vi "Puff_using_Arduino.vi"() -> (5 "Plug in titles":string[](array[string]), 7 "Plug in values":string[](array[string]))   [LabVIEW 2013]
uses:
  Controls/Post_Process.ctl
  Controls/Setup.ctl
  Globals/Meas_global.vi
panel:
  out "Puff Time used":dbl=1.0 format="%.2g"
  out "EnFlo_Tunnel Metadata:Puff_duration:Sec":dbl=1.0 format="%.2g"
  out "Case Currently On":string="Loop"
  # "Change this value via the ADAM Scan Table"
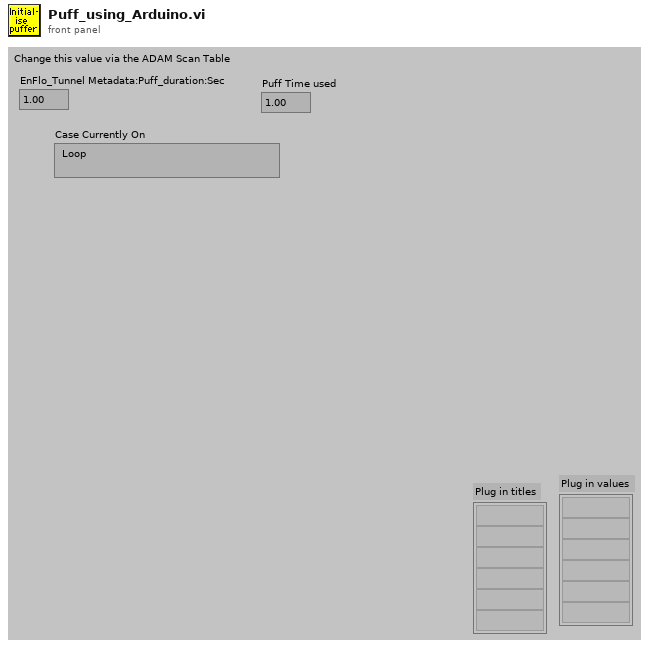
[diagram p1: front panel]
types:
  T1 = typedef "Setup.ctl" = enum16{"Run Program", "Show Setup", "Save Current Setup", "Setup Front Panel"}
  T2 = typedef "Post_Process.ctl" = enum16{"Take New Data", "Post Process Raw Data File"}
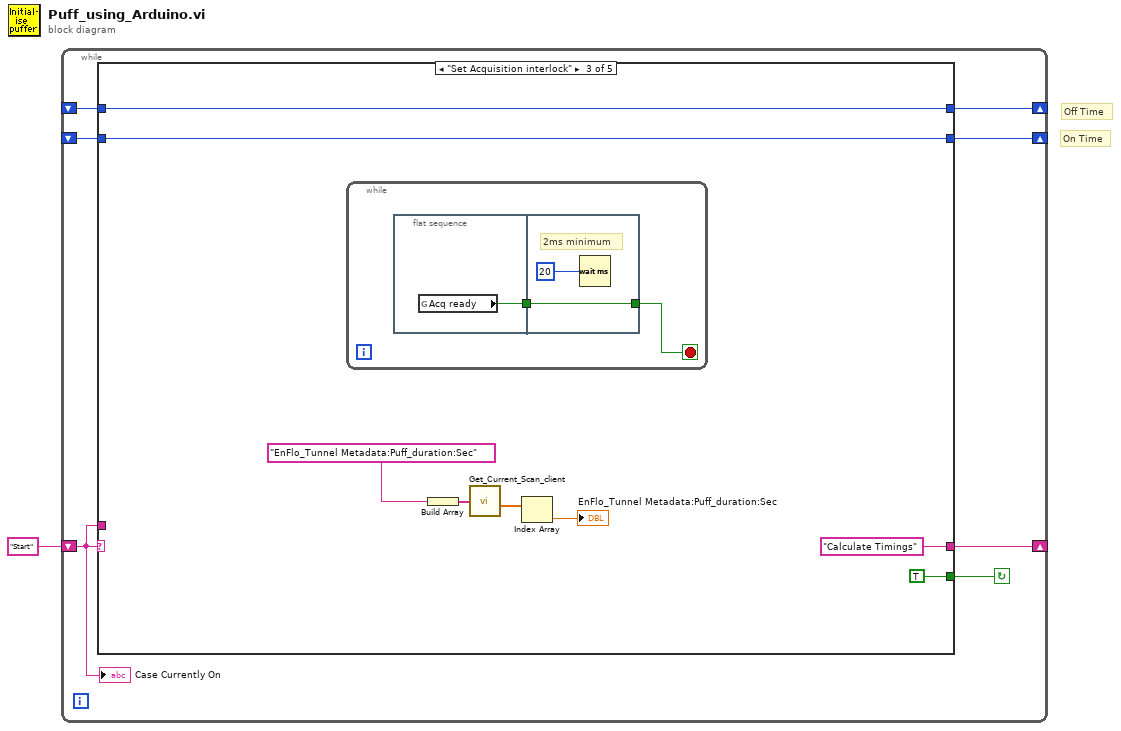
[diagram p0: block diagram]
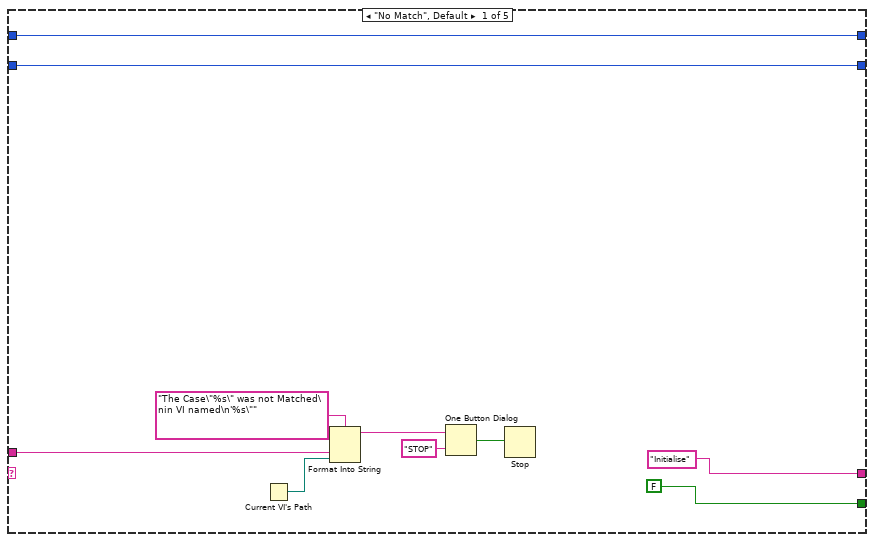
[diagram p2: hidden frame]
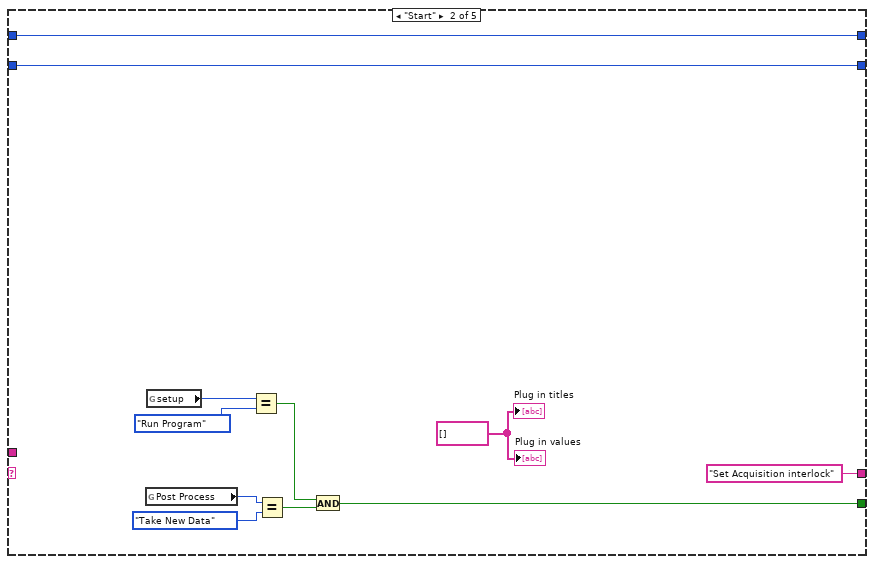
[diagram p3: hidden frame]
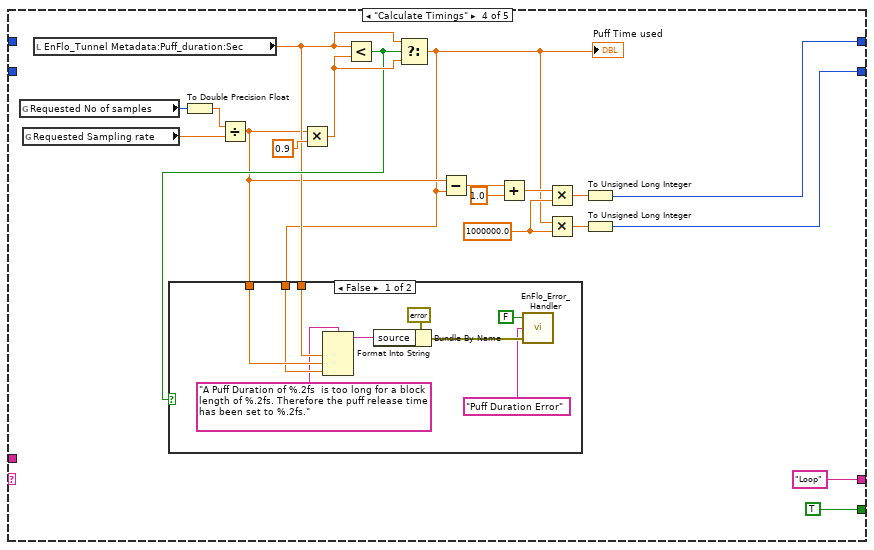
[diagram p4: hidden frame]
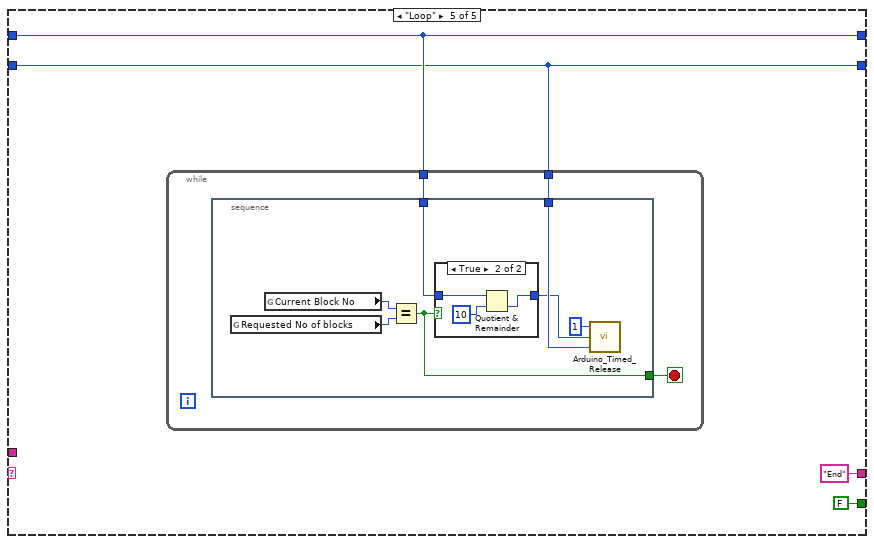
[diagram p6: hidden frame]
diagram:
  # "On Time"
  # "Off Time"
  n1 = while {
    shift-left: "Start" -> [w6]
    shift-right: [w7] -> _
    shift-right: [w5] -> _
    shift-left: _ -> [w4]
    shift-right: [w3] -> _
    shift-left: _ -> [w2]
    stop <- w8 continue-if-true
    n2 = case shown="\"Set Acquisition interlock\"" w6 {
      tunnel: [FALSE w21 TRUE ("Command Found") TRUE ("Command Found") FALSE ("Command Found")] -> w8
      tunnel: ["Initialise" "Set Acquisition interlock" "Calculate Timings" "Loop" "End"] -> w7
      tunnel: w6 -> [w13 _ _ _ _]
      tunnel: [w10 w20 w31 w45 w74] -> w5
      tunnel: w4 -> [w10 w20 w31 _ w74]
      tunnel: [w9 w19 w30 w44 w73] -> w3
      tunnel: w2 -> [w9 w19 w30 _ w73]
      frame "No Match", Default {
        n3 = Current VI's Path() -> (path=w12:path)
        n4 = Format Into String(format string="The Case\"%s\" was not Matched\nin VI named\n'%s\"" ("Format String"), w13, w12) -> (resulting string=w16:string)  [unwired: 2 in, 1 out]
        n5 = One Button Dialog(message=w16, button name ("OK")="STOP") -> (true=w14:bool)
        n6 = Stop(stop? (T)=w14) -> ()
      }
      frame "Start" {
        w28 = string[] [] ("Plug in titles")
        n7 = global read "Meas_global.vi" "Post Process"() -> (w23:T2)
        n8 = global read "Meas_global.vi" "setup"() -> (w22:T1)
        n9 = Equal?(x=w22, y=Setup."Run Program") -> (x = y?=w27:bool)
        n10 = Equal?(x=w23, y=Post_Process."Take New Data" ("Post Process")) -> (x = y?=w26:bool)
        n11 = And(x=w27, y=w26) -> (x .and. y?=w21:bool)
        "Plug in values" <- w28
        "Plug in titles" <- w28
      }
      frame "Set Acquisition interlock" {
        n12 = while {
          stop <- w39 stop-if-true
          n13 = flat-sequence {
            tunnel: [w40] -> w38
            tunnel: [w42] -> w39
            tunnel: w38 -> [w42]
            frame #0 {
              n14 = global read "Meas_global.vi" "Acq ready"() -> (w40:bool)
            }
            frame #1 {
              # "2ms minimum"
              n15 = Wait (ms)(milliseconds to wait=u32 20) -> ()  [unwired: 1 out]
            }
          }
        }
        n16 = Build Array("EnFlo_Tunnel Metadata:Puff_duration:Sec") -> (w34:string[])
        n17 = call "Get_Current_Scan_client.vi"("ADAM Ch Names"=w34) -> ("Numerical Values"=w33:dbl[])  [unwired: 1 in, 2 out]
        n18 = Index Array(array=w33) -> (element=→"EnFlo_Tunnel Metadata:Puff_duration:Sec":dbl)  [unwired: 1 in]
      }
      frame "Calculate Timings" {
        w54 = 1000000.0 ("y")
        n19 = global read "Meas_global.vi" "Requested No of samples"() -> (w59:i32)
        n20 = global read "Meas_global.vi" "Requested Sampling rate"() -> (w48:dbl)
        n21 = local read "EnFlo_Tunnel Metadata:Puff_duration:Sec"() -> (w49:dbl)
        n22 = To Double Precision Float(number=w59) -> (double precision float=w43:dbl)
        n23 = Divide(x=w43, y=w48) -> (x/y=w47:dbl)
        n24 = Multiply(x=w47, y=0.9) -> (x*y=w57:dbl)
        n25 = Less?(x=w49, y=w57) -> (x < y?=w50:bool)
        n26 = Select(t=w49, s=w50, f=w57) -> (s? t:f=w46:dbl)
        "Puff Time used" <- w46
        n27 = case shown="False" w50 {
          tunnel: w49 -> [w68 _]
          tunnel: w47 -> [w67 _]
          tunnel: w46 -> [w66 _]
          frame False {
            n28 = Format Into String(format string="A Puff Duration of %.2fs  is too long for a block length of %.2fs. Therefore the puff release time has been set to %.2fs.", w68, w67, w66) -> (resulting string=w64:string)  [unwired: 2 in, 1 out]
            n29 = Bundle By Name(cluster=errorcluster {"status"=TRUE, "code"=0, "source"=""} ("error in (no error)"), "source"=w64) -> (w69:errorcluster)
            n30 = call "EnFlo_Error_Handler.vi"("error in (no error)"=w69, "Error Type"="Puff Duration Error", "Dialog Box (T)"=FALSE) -> ()  [unwired: 3 out]
          }
          frame True {
          }
        }
        n31 = Subtract(x=w47, y=w46) -> (x-y=w53:dbl)
        n32 = Add(x=w53, y=1.0) -> (x+y=w51:dbl)
        n33 = Multiply(x=w51, y=w54) -> (x*y=w55:dbl)
        n34 = Multiply(x=w46, y=w54) -> (x*y=w56:dbl)
        n35 = To Unsigned Long Integer(number=w55) -> (unsigned 32bit integer=w45:u32)
        n36 = To Unsigned Long Integer(number=w56) -> (unsigned 32bit integer=w44:u32)
      }
      frame "Loop" {
        n37 = while {
          tunnel: w74 -> [w75]
          tunnel: w73 -> [w77]
          stop <- w76 stop-if-true
          n38 = stacked-sequence {
            tunnel: w77 -> [w83]
            tunnel: [w78] -> w76
            tunnel: w75 -> [w82]
            frame #0 {
              n39 = global read "Meas_global.vi" "Requested No of blocks"() -> (w80:i32)
              n40 = global read "Meas_global.vi" "Current Block No"() -> (w79:i32)
              n41 = Equal?(x=w79, y=w80) -> (x = y?=w78:bool)
              n42 = case shown="True" w78 {
                tunnel: w82 -> [w85 w88]
                tunnel: [w85 w86] -> w81
                frame False {
                }
                frame True {
                  n43 = Quotient & Remainder(x=w88, y=u32 10) -> (floor(x/y)=w86:u32)  [unwired: 1 out]
                }
              }
              n44 = call "Arduino_Timed_Release.vi"("Time to hold source ON (microseconds)"=w83, "Time to hold source OFF (microseconds)"=w81, "Number of cycles"=u16 1) -> ()  [unwired: 2 out]
            }
          }
        }
      }
    }
    "Case Currently On" <- w6
  }
